vi "Generate Controls for Client.vi"(8 "error in":errorcluster, 9 "control name":string, 10 "parameter data":T1[](array[typedef]), 11 "measure vi refnum":refnum<vi>) -> (0 "error out":errorcluster, 2 "control refnum":refnum<vi>, 3 "measure vi refnum out":refnum<vi>)   [LabVIEW 2021, in "MeasurementClient Editor.lvlib"]
uses:
  <vilib>/gRPC/Generated APIs/ni/measurementlink/measurement/v2/RPC Messages/ni_measurementlink_measurement_v2_ConfigurationParameter.ctl
  <vilib>/gRPC/Generated APIs/ni/measurementlink/measurement/v2/RPC Messages/google_protobuf_Field_Kind.ctl
  <vilib>/gRPC/Generated APIs/ni/measurementlink/measurement/v2/RPC Messages/ni_measurementlink_measurement_v2_ConfigurationParameter_AnnotationsEntry.ctl
  MeasurementClient Editor.lvlib
  <vilib>/gRPC/Generated APIs/ni/measurementlink/measurement/v2/ni.measurementlink.measurement.v2.api.lvlib
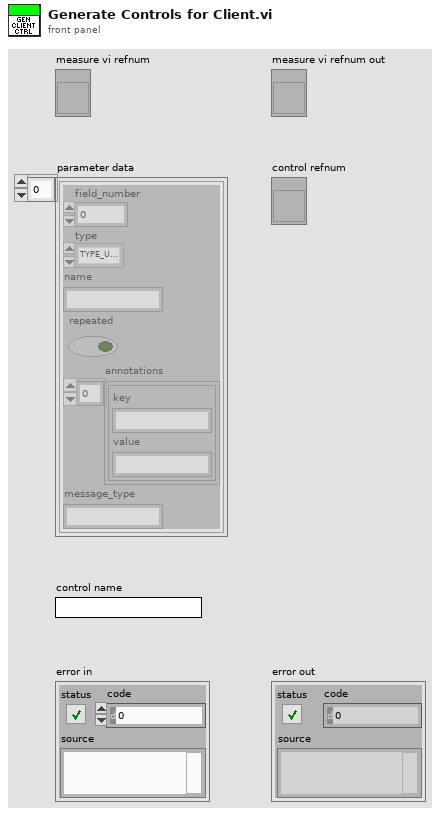
[diagram p1: front panel]
types:
  T1 = typedef "ni.measurementlink.measurement.v2.api.lvlib/ni_measurementlink_measurement_v2_ConfigurationParameter.ctl" = cluster{"field_number":i32, "type":T2, "name":string, "repeated":bool, "annotations":T3[], "message_type":string}
  T2 = typedef "ni.measurementlink.measurement.v2.api.lvlib/google_protobuf_Field_Kind.ctl" = enum32{"TYPE_UNKNOWN", "TYPE_DOUBLE", "TYPE_FLOAT", "TYPE_INT64", "TYPE_UINT64", "TYPE_INT32", "TYPE_FIXED64", "TYPE_FIXED32", "TYPE_BOOL", "TYPE_STRING", "TYPE_GROUP", "TYPE_MESSAGE", "TYPE_BYTES", "TYPE_UINT32", "TYPE_ENUM", "TYPE_SFIXED32", "TYPE_SFIXED64", "TYPE_SINT32", "TYPE_SINT64"}
  T3 = typedef "ni.measurementlink.measurement.v2.api.lvlib/ni_measurementlink_measurement_v2_ConfigurationParameter_AnnotationsEntry.ctl" = cluster{"key":string, "value":string}
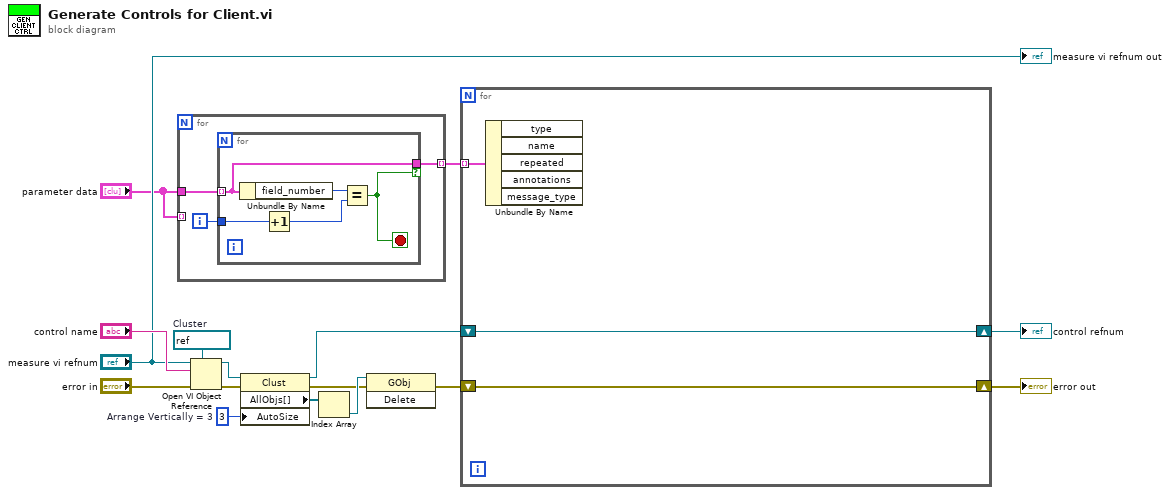
[diagram p0: block diagram]
diagram:
  w7 = u32 3  # Arrange Vertically = 3
  w16 = refnum<vi> refnum  # Cluster
  n1 = for {
    tunnel: "parameter data" -> [w19]
    tunnel: [w17] -> w1 mode=indexing
    tunnel: "parameter data" -> [_] mode=indexing
    i -> [w18]
    n2 = for {
      tunnel: w19 -> [w21] mode=indexing
      tunnel: w18 -> [w24]
      tunnel: [w21] -> w17 if=w20
      stop <- w20 stop-if-true
      n3 = Unbundle By Name(w21) -> ("field_number"=w23:i32)
      n4 = Increment(x=w24) -> (x+1=w22:i32)
      n5 = Equal?(x=w23, y=w22) -> (x = y?=w20:bool)
    }
  }
  n6 = Open VI Object Reference(7:w16, 8:"error in", 10:"control name", 11:"measure vi refnum") -> (0:w14:errorcluster, 3:w15:refnum<vi>)
  n7 = property class="Clust"(reference=w15, error in=w14, "AutoSize"=w7) -> (reference out=w5:refnum<vi>, error out=w11:errorcluster, "AllObjs[]"=w13:refnum<vi>[])
  n8 = Index Array(array=w13) -> (element=w12:refnum<vi>)  [unwired: 1 in]
  n9 = invoke class="GObj" method="Delete"(reference=w12, error in=w11) -> (error out=w6:errorcluster)  [unwired: 1 in, 2 out]
  n10 = for {
    tunnel: w1 -> [w25] mode=indexing
    shift-right: [w27] -> w3
    shift-left: w5 -> [w27]
    shift-right: [w26] -> w4
    shift-left: w6 -> [w26]
    n11 = Unbundle By Name(w25) -> ()  [unwired: 5 out]
  }
  "error out" <- w4
  "control refnum" <- w3
  "measure vi refnum out" <- "measure vi refnum"
